vi "Control Panel Edit.vi"(10 "Project":string, 11 "Data In":string[][](array[string])) -> (2 "OK?":bool, 3 "Data Out":string[][](array[string]))   [LabVIEW 2020]
panel:
  in  "Data":cluster{"ID":string, "Name":string}[](array[cluster])
  in  "Cancel":bool
  in  "OK":bool
  # "标识符"
  # "名称"
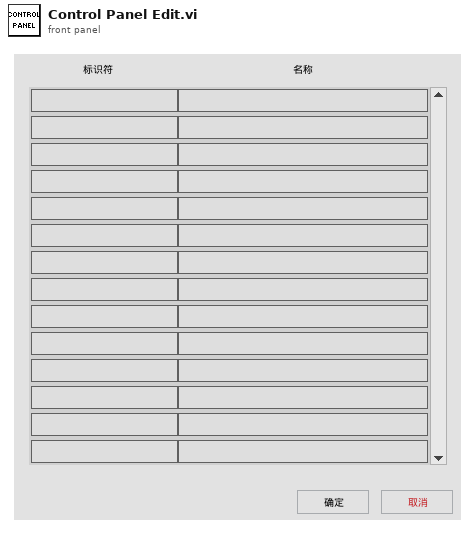
[diagram p1: front panel]
types:
  T1 = typedef "LVPoint32TypeDef.ctl" = cluster{"Horizontal":i32, "Vertical":i32}
  T2 = cluster{"Data":cluster{"ID":string, "Name":string}[], "Project":string, "OK?":bool, "Data Out":string[][]}
  T3 = typedef "SDQ Data Type.ctl" = cluster{"CAN Length":string, "CAN Name":string, "CAN ID":string, "CAN Type":string, "Test Item":string, "Byte Order":string, "Instruction":string, "Control Type":string, "Group":string, "Offset":dbl, "Coefficient":dbl, "Write Enable":bool, "Lable Type":string, "Key?":string, "Set Value":string, "Upper":dbl, "Lower":dbl, "Unit":string, "Formula":string, "Test Item Type":string, "Length":i32, "Address":string, "Name":string, "Identifier":string, "Data Type":string, "Enumerate?":string, "Enumerate List":string, "Data":string, "Source":string}
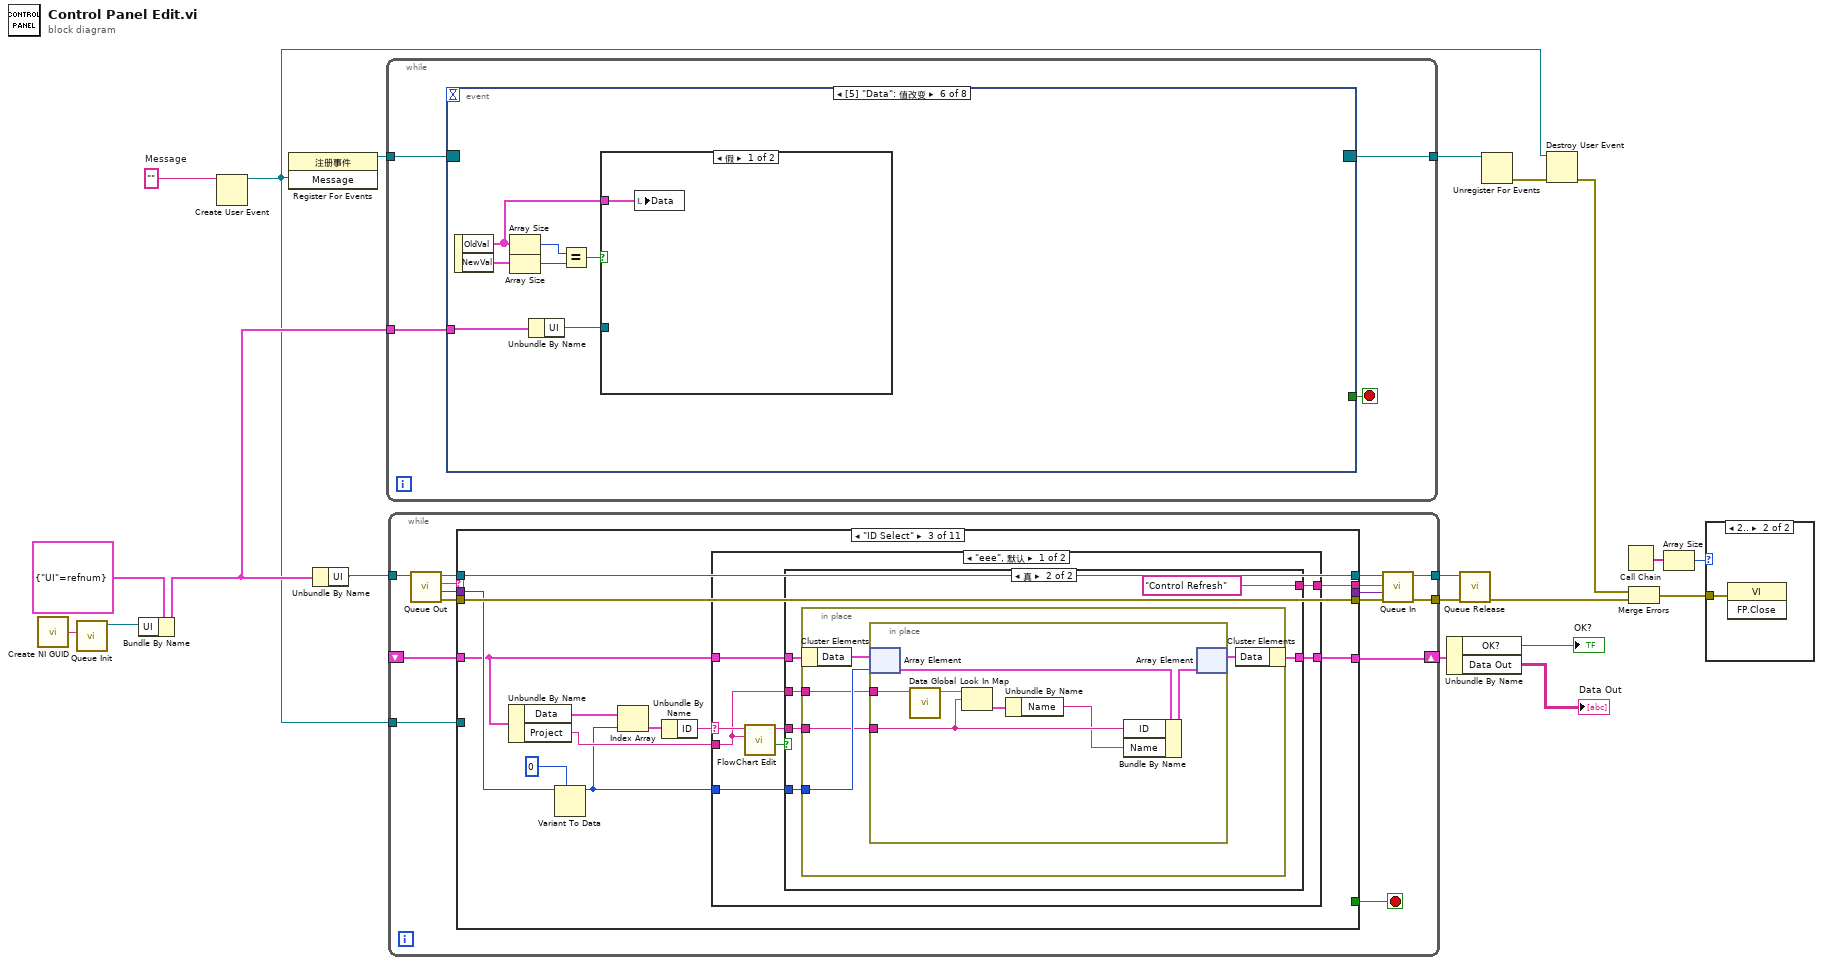
[diagram p0: block diagram]
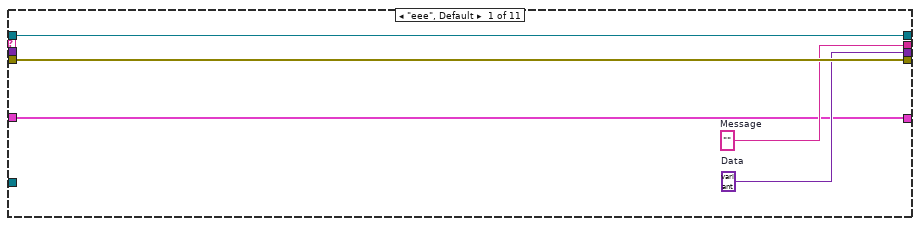
[diagram p3: hidden frame]
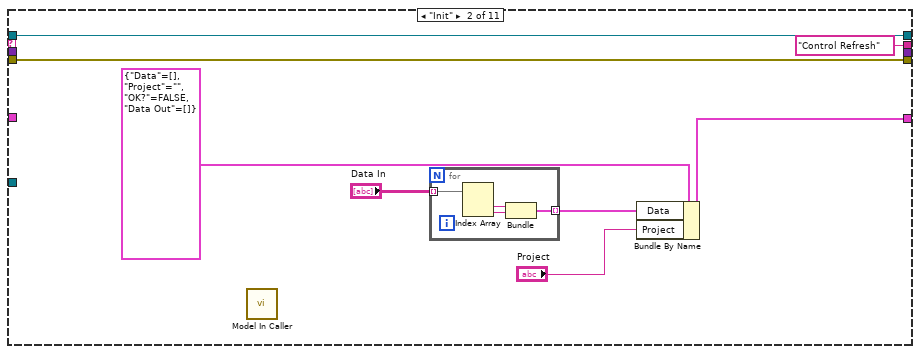
[diagram p4: hidden frame]
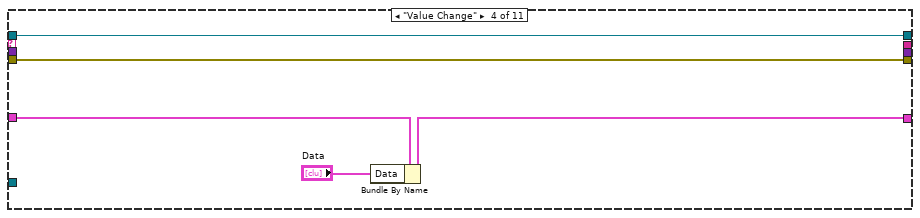
[diagram p7: hidden frame]
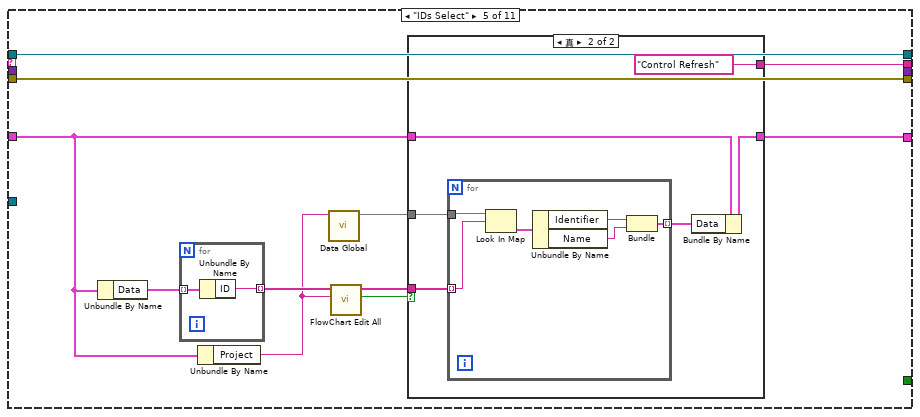
[diagram p8: hidden frame]
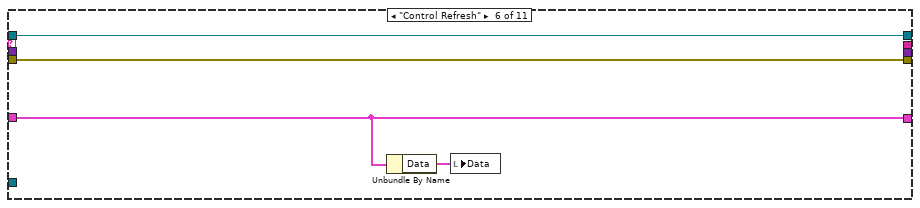
[diagram p10: hidden frame]
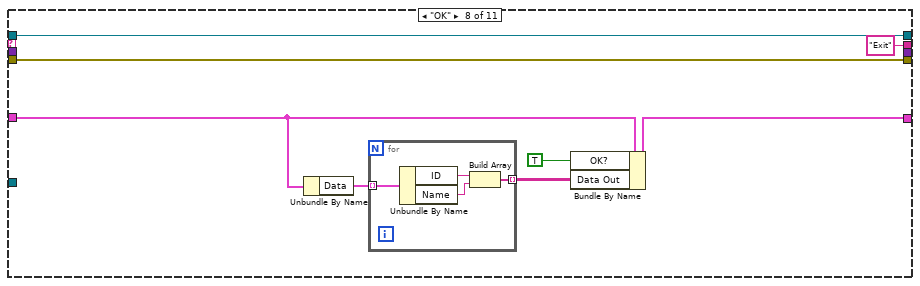
[diagram p12: hidden frame]
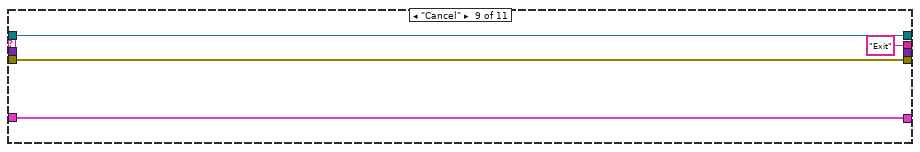
[diagram p13: hidden frame]
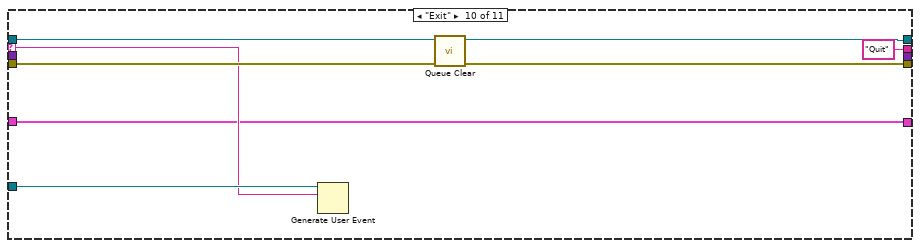
[diagram p14: hidden frame]
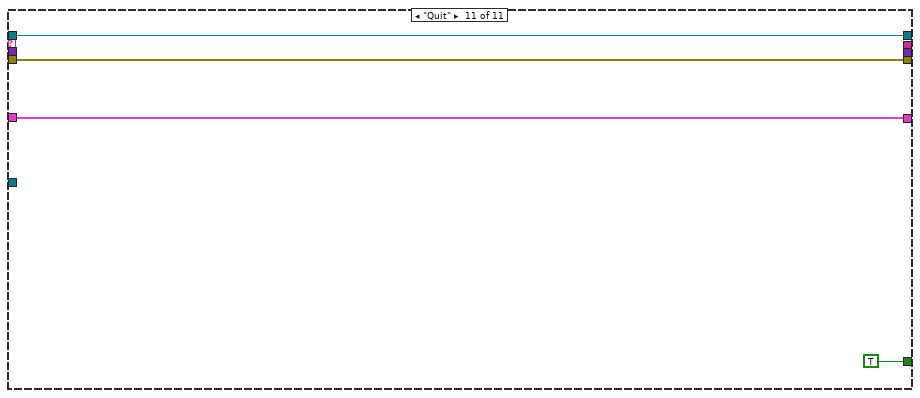
[diagram p15: hidden frame]
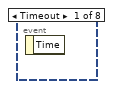
[diagram p16: hidden frame]
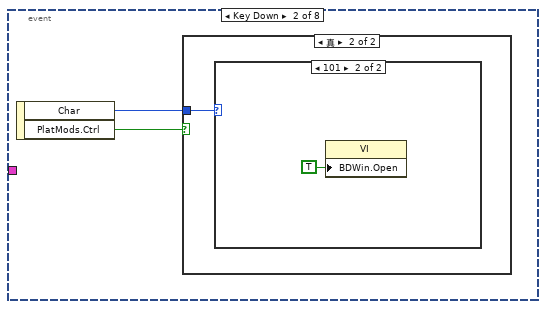
[diagram p17: hidden frame]
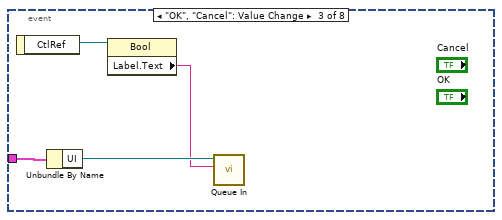
[diagram p20: hidden frame]
diagram:
  w16 = ""  # Message
  n1 = call <vilib>:"Create NI GUID.vi"() -> ("NI GUID"=w18:string)
  n2 = call "Queue Init.vi"("Queue Name"=w18) -> ("Queue Out"=w20:refnum<queue>)  [unwired: 8 in, 2 out]
  n3 = Bundle By Name(cluster=cluster{"UI":refnum<queue>} {"UI"=refnum} ("Queue Ref Out"), "UI"=w20) -> (w19:cluster{"UI":refnum<queue>})
  n4 = Create User Event(user event datatype=w16) -> (user event=w12:refnum<user-event>)  [unwired: 1 in, 1 out]
  n5 = register-events(w12) -> (reference out=w15:refnum<event-registration>)  [unwired: 2 in, 1 out]
  n6 = Unbundle By Name(w19) -> ("UI"=w9:refnum<queue>)
  n7 = while {
    tunnel: w15 -> [w24]
    tunnel: [w22] -> w14
    tunnel: w19 -> [w21]
    stop <- w23 stop-if-true
    n8 = event shown="[5] \"Data\": 值改变" {
      selector: w24 -> [_ _ _ _ _ _ _ _]
      dyn-events: [_ _ _ _ _ _ _ _] -> w22
      timeout: _ -> [_ _ _ _ _ _ _ _]
      tunnel: [_ _ _ _ _ _ w69 _] -> w23
      tunnel: w21 -> [_ _ w32 w35 w44 w61 _ w74]
      event Timeout {
        n9 = event-data() -> ()  [unwired: 1 in, 1 out]
      }
      event Key Down {
        n10 = event-data() -> ("Char"=w26:i16, "PlatMods.Ctrl"=w25:bool)  [unwired: 1 in]
        n11 = case shown="真" w25 {
          tunnel: w26 -> [_ w27]
          frame False {
          }
          frame True {
            n12 = case shown="101" w27 {
              frame 0, Default {
              }
              frame 101 {
                n13 = property class="VI"("BDWin.Open"=TRUE ("程序框图窗口:打开")) -> ()  [unwired: 2 in, 2 out]
              }
            }
          }
        }
      }
      event "OK", "Cancel": Value Change {
        n14 = event-data() -> ("CtlRef"=w30:refnum<vi>)  [unwired: 1 in]
        n15 = Unbundle By Name(w32) -> ("UI"=w31:refnum<queue>)
        n16 = property class="Bool"(reference=w30) -> ("Label.Text"=w29:string)  [unwired: 1 in, 2 out]
        n17 = call "Queue In.vi"("Message"=w29, "Queue In"=w31) -> ()  [unwired: 8 in, 2 out]
      }
      event Panel Resize {
        n18 = event-data() -> ()  [unwired: 1 in, 1 out]
        n19 = Unbundle By Name(w35) -> ("UI"=w34:refnum<queue>)
        n20 = call "Queue In.vi"("Message"="Panel Change", "Queue In"=w34) -> ()  [unwired: 8 in, 2 out]
      }
      event "Data": Mouse Down {
        n21 = event-data() -> ("Mods.Double Click"=w52:bool, "CtlRef"=w51:refnum<vi>, "Coords"=w50:T1)  [unwired: 1 in]
        n22 = property class="Arr (严格)"(reference=w51) -> ("Top"=w49:i32, "Array Element.Height"=w46:u32, "Index Values"=w38:u32[])  [unwired: 1 in, 2 out]
        n23 = Unbundle By Name(w50) -> ("Vertical"=w48:i32, "Horizontal"=w41:i32)
        n24 = Subtract(x=w48, y=w49) -> (x-y=w47:i32)
        n25 = Divide(x=w47, y=w46) -> (x/y=w45:dbl)
        n26 = Index Array(array=w38) -> (element=w37:u32)  [unwired: 1 in]
        n27 = Round Toward -Infinity(1:w45) -> (0:w36:dbl)
        n28 = Add(x=w37, y=w36) -> (x+y=w40:dbl)
        n29 = To Unsigned Long Integer(number=w40) -> (unsigned 32bit integer=w39:u32)
        n30 = case shown="假" w52 {
          tunnel: [w53 "IDs Select" ("Message")] -> w42
          tunnel: w41 -> [w56 _]
          frame False {
            n31 = property on="Name" class="Str"() -> ("Left"=w55:i32)  [unwired: 2 in, 2 out]
            n32 = Less?(x=w56, y=w55) -> (x < y?=w54:bool)
            n33 = case shown="真" w54 {
              tunnel: [_ "ID Select"] -> w53
              frame False {
              }
              frame True {
              }
            }
          }
          frame True {
          }
        }
        n34 = Unbundle By Name(w44) -> ("UI"=w43:refnum<queue>)
        n35 = call "Queue In.vi"("Data"=w39, "Message"=w42, "Queue In"=w43) -> ()  [unwired: 7 in, 2 out]
      }
      event "Data": Value Change {
        n36 = event-data() -> ("OldVal"=w59:cluster{"ID":string, "Name":string}[], "NewVal"=w65:cluster{"ID":string, "Name":string}[])  [unwired: 1 in]
        n37 = Array Size(array=w59) -> (size(s)=w64:i32)
        n38 = Array Size(array=w65) -> (size(s)=w63:i32)
        n39 = Unbundle By Name(w61) -> ("UI"=w60:refnum<queue>)
        n40 = Equal?(x=w64, y=w63) -> (x = y?=w62:bool)
        n41 = case shown="假" w62 {
          tunnel: w60 -> [_ w68]
          tunnel: w59 -> [w66 _]
          frame False {
            n42 = local write "Data"(w66) -> ()
          }
          frame True {
            n43 = call "Queue In.vi"("Message"="Value Change", "Queue In"=w68) -> ()  [unwired: 8 in, 2 out]
          }
        }
      }
      event User Event {
        n44 = event-data() -> ("Message"=w71:string)  [unwired: 1 in]
        n45 = Equal?(x=w71, y="Exit") -> (x = y?=w69:bool)
      }
      event Panel Close? {
        n46 = event-data() -> ()  [unwired: 1 in, 1 out]
        n47 = Unbundle By Name(w74) -> ("UI"=w73:refnum<queue>)
        n48 = call "Queue In.vi"("Message"="Exit", "Queue In"=w73) -> ()  [unwired: 8 in, 2 out]
        n49 = event-data("Discard?"=TRUE ("放弃？")) -> ()  [unwired: 1 in, 1 out]
      }
    }
  }
  n50 = while {
    tunnel: w9 -> [w85]
    tunnel: [w82] -> w11
    tunnel: [w81] -> w10
    tunnel: w12 -> [w89]
    shift-right: [w77] -> w3
    shift-left: _ -> [w76]
    stop <- w90 stop-if-true
    n51 = call "Queue Out.vi"("Queue In"=w85) -> ("error out"=w88:errorcluster, "Data"=w86:variant, "Message"=w87:string, "Queue Out"=w84:refnum<queue>)  [unwired: 6 in, 1 out]
    n52 = case shown="\"ID Select\"" w87 {
      selector: w87 -> [_ _ _ _ _ _ _ _ _ w203 _]
      tunnel: w84 -> [w95 w103 w119 w152 w163 w182 w185 w193 w201 w207 w212]
      tunnel: w88 -> [w94 w102 w118 w151 w162 w181 w184 w192 w200 w205 w213]
      tunnel: [w95 w103 w119 w152 w163 w182 w185 w193 w201 w206 w212] -> w83
      tunnel: [w94 w102 w118 w151 w162 w181 w184 w192 w200 w204 w213] -> w80
      tunnel: [w93 "Control Refresh" ("Message") w108 _ w153 _ _ "Exit" ("Message") "Exit" ("Message") "Quit" _] -> w79
      tunnel: [_ _ _ _ _ _ _ _ _ _ TRUE] -> w90
      tunnel: w89 -> [_ _ _ _ _ _ _ _ _ w209 _]
      tunnel: [w92 _ _ _ _ _ _ _ _ _ _] -> w78
      tunnel: w86 -> [_ _ w116 _ _ _ _ _ _ _ _]
      tunnel: [w91 w99 w111 w149 w155 w180 w183 w190 w198 w202 w210] -> w77
      tunnel: w76 -> [w91 _ w112 w150 w160 w180 w183 w188 w198 w202 w210]
      frame "eee", Default {
        w92 = variant  # Data
        w93 = ""  # Message
      }
      frame "Init" {
        n53 = call "Model In Caller.vi"() -> ()  [unwired: 11 in, 1 out]
        n54 = for {
          tunnel: "Data In" -> [w107] mode=indexing
          tunnel: [w104] -> w97 mode=indexing
          n55 = Index Array(array=w107) -> (element #1=w106:string, element #2=w105:string)  [unwired: 2 in]
          n56 = Bundle("字符串"=w106, "字符串"=w105) -> (w104:cluster{"字符串":string, "字符串":string})  [unwired: 1 in]
        }
        n57 = Bundle By Name(cluster=T2 {"Data"=[], "Project"="", "OK?"=FALSE, "Data Out"=[]}, "Data"=w97, "Project"="Project") -> (w99:T2)
      }
      frame "ID Select" {
        n58 = Unbundle By Name(w112) -> ("Data"=w117:cluster{"ID":string, "Name":string}[], "Project"=w113:string)
        n59 = Variant To Data(type=u32 0 ("无符号32位整型"), Variant=w116) -> (data=w110:u32)  [unwired: 1 in, 1 out]
        n60 = Index Array(array=w117, index=w110) -> (element=w114:cluster{"ID":string, "Name":string})
        n61 = Unbundle By Name(w114) -> ("ID"=w109:string)
        n62 = case shown="\"eee\", 默认" w109 {
          selector: w109 -> [w127 _]
          tunnel: w113 -> [w122 _]
          tunnel: w112 -> [w126 w147]
          tunnel: [w125 w147] -> w111
          tunnel: w110 -> [w124 _]
          tunnel: [w120 _] -> w108
          frame "eee", Default {
            n63 = call "FlowChart Edit.vi"("Name"=w122, "Identifier In"=w127) -> ("OK？"=w121:bool, "Identifier Out"=w123:string)  [unwired: 6 in, 2 out]
            n64 = case shown="真" w121 {
              tunnel: w126 -> [w128 w134]
              tunnel: [w128 w133] -> w125
              tunnel: w124 -> [_ w132]
              tunnel: w123 -> [_ w131]
              tunnel: w122 -> [_ w130]
              tunnel: [_ "Control Refresh"] -> w120
              frame False {
              }
              frame True {
                n65 = in-place {
                  in-place-border: w132 -> [w138]
                  in-place-border: w131 -> [w136]
                  in-place-border: w130 -> [w135]
                  n66 = in-place-cluster #1(w134) -> ("Data"=w139:cluster{"ID":string, "Name":string}[])
                  n67 = in-place {
                    in-place-border: w136 -> [w142]
                    in-place-border: w135 -> [w144]
                    n68 = in-place-array #2(w139, w138) -> (w146:cluster{"ID":string, "Name":string})
                    n69 = call "Data Global.vi"("Name"=w144) -> ("Data Out"=w143:map{string, T3})  [unwired: 7 in, 3 out]
                    n70 = Look In Map(map=w143, key=w142) -> (value=w141:T3)  [unwired: 1 in, 1 out]
                    n71 = Unbundle By Name(w141) -> ("Name"=w140:string)
                    n72 = Bundle By Name(cluster=w146, "ID"=w142, "Name"=w140) -> (w145:cluster{"ID":string, "Name":string})
                    n73 = in-place-array #2(w145) -> (w137:cluster{"ID":string, "Name":string}[])  [unwired: 1 out]
                  }
                  n74 = in-place-cluster #1("Data"=w137) -> (w133:T2)
                }
              }
            }
          }
          frame "" {
          }
        }
      }
      frame "Value Change" {
        n75 = Bundle By Name(cluster=w150, "Data"="Data") -> (w149:T2)
      }
      frame "IDs Select" {
        n76 = Unbundle By Name(w160) -> ("Data"=w161:cluster{"ID":string, "Name":string}[])
        n77 = for {
          tunnel: w161 -> [w178] mode=indexing
          tunnel: [w177] -> w159 mode=indexing
          n78 = Unbundle By Name(w178) -> ("ID"=w177:string)
        }
        n79 = Unbundle By Name(w160) -> ("Project"=w158:string)
        n80 = call "Data Global.vi"("Name"=w158) -> ("Data Out"=w157:map{string, T3})  [unwired: 7 in, 3 out]
        n81 = call "FlowChart Edit All.vi"("Name"=w158, "Identifier In"=w159) -> ("OK？"=w154:bool, "Identifiers Out"=w156:string[])  [unwired: 8 in]
        n82 = case shown="真" w154 {
          tunnel: w160 -> [w164 w170]
          tunnel: w157 -> [_ w169]
          tunnel: w156 -> [_ w168]
          tunnel: [w164 w167] -> w155
          tunnel: [_ "Control Refresh" ("Message")] -> w153
          frame False {
          }
          frame True {
            n83 = for {
              tunnel: w169 -> [w176]
              tunnel: w168 -> [w175] mode=indexing
              tunnel: [w171] -> w166 mode=indexing
              n84 = Look In Map(map=w176, key=w175) -> (value=w174:T3)  [unwired: 1 in, 1 out]
              n85 = Unbundle By Name(w174) -> ("Identifier"=w173:string, "Name"=w172:string)
              n86 = Bundle("Identifier"=w173, "Name"=w172) -> (w171:cluster{"Identifier":string, "Name":string})  [unwired: 1 in]
            }
            n87 = Bundle By Name(cluster=w170, "Data"=w166) -> (w167:T2)
          }
        }
      }
      frame "Control Refresh" {
        n88 = Unbundle By Name(w180) -> ("Data"=w179:cluster{"ID":string, "Name":string}[])
        n89 = local write "Data"(w179) -> ()
      }
      frame "Panel Change" {
      }
      frame "OK" {
        n90 = Unbundle By Name(w188) -> ("Data"=w187:cluster{"ID":string, "Name":string}[])
        n91 = for {
          tunnel: w187 -> [w197] mode=indexing
          tunnel: [w194] -> w186 mode=indexing
          n92 = Unbundle By Name(w197) -> ("ID"=w196:string, "Name"=w195:string)
          n93 = Build Array(w196, w195) -> (w194:string[])
        }
        n94 = Bundle By Name(cluster=w188, "OK?"=TRUE, "Data Out"=w186) -> (w190:T2)
      }
      frame "Cancel" {
      }
      frame "Exit" {
        n95 = Generate User Event(user event=w209, event data cluster=w203) -> ()  [unwired: 2 in, 2 out]
        n96 = call "Queue Clear.vi"("error in (no error)"=w205, "Queue In"=w207) -> ("error out"=w204:errorcluster, "Queue Out"=w206:refnum<queue>)  [unwired: 8 in]
      }
      frame "Quit" {
      }
    }
    n97 = call "Queue In.vi"("error in (no error)"=w80, "Data"=w78, "Message"=w79, "Queue In"=w83) -> ("error out"=w81:errorcluster, "Queue Out"=w82:refnum<queue>)  [unwired: 6 in]
  }
  n98 = Unbundle By Name(w3) -> ("OK?"=→"OK?":bool, "Data Out"=→"Data Out":string[][])
  n99 = call "Queue Release.vi"("error in (no error)"=w10, "Queue In"=w11) -> ("error out"=w7:errorcluster)  [unwired: 9 in]
  n100 = Unregister For Events(event registration refnum=w14) -> (error out=w13:errorcluster)  [unwired: 1 in]
  n101 = Destroy User Event(user event=w12, error in=w13) -> (error out=w8:errorcluster)
  n102 = Call Chain() -> (call chain=w5:string[])
  n103 = Merge Errors(w8, w7) -> (w6:errorcluster)
  n104 = Array Size(array=w5) -> (size(s)=w4:i32)
  n105 = case shown="2.." w4 {
    tunnel: w6 -> [_ w214]
    frame 0, Default {
    }
    frame 2.. {
      n106 = invoke class="VI" method="FP.Close"(error in=w214) -> ()  [unwired: 2 in, 3 out]
    }
  }
